vi "Get Challenge Config By Id.vi"(8 "Error In":errorcluster, 11 "VIChallenge Config":T2) -> (0 "Error Out":errorcluster, 2 "Challenge Config":T1, 3 "VIChallenge Config":T2)   [LabVIEW 2013, in "VIChallenge.lvlib"]
uses:
  VIChallenge.lvlib
  Type Defs/VIChallenge Config.ctl
  <vilib>/National Instruments/NI Amazon Web Services (AWS) Toolkit for LabVIEW/SQS/VI Source/AWS SQS Class/AWS_SQS.lvclass
  <vilib>/National Instruments/NI Amazon Web Services (AWS) Toolkit for LabVIEW/AWS Core Lib/VI Source/Typedefs/AWS_AWS Credentials.ctl
  Type Defs/JSON_job.ctl
  <vilib>/addons/database/Connection.llb/Conn ObjectReference.ctl
  Grader/Type Defs/Challenge.ctl
  <vilib>/National Instruments/NI Amazon Web Services (AWS) Toolkit for LabVIEW/AWS Core Lib/VI Source/AWS_Core.lvlib
  <vilib>/addons/database/NI_Database_API.lvlib
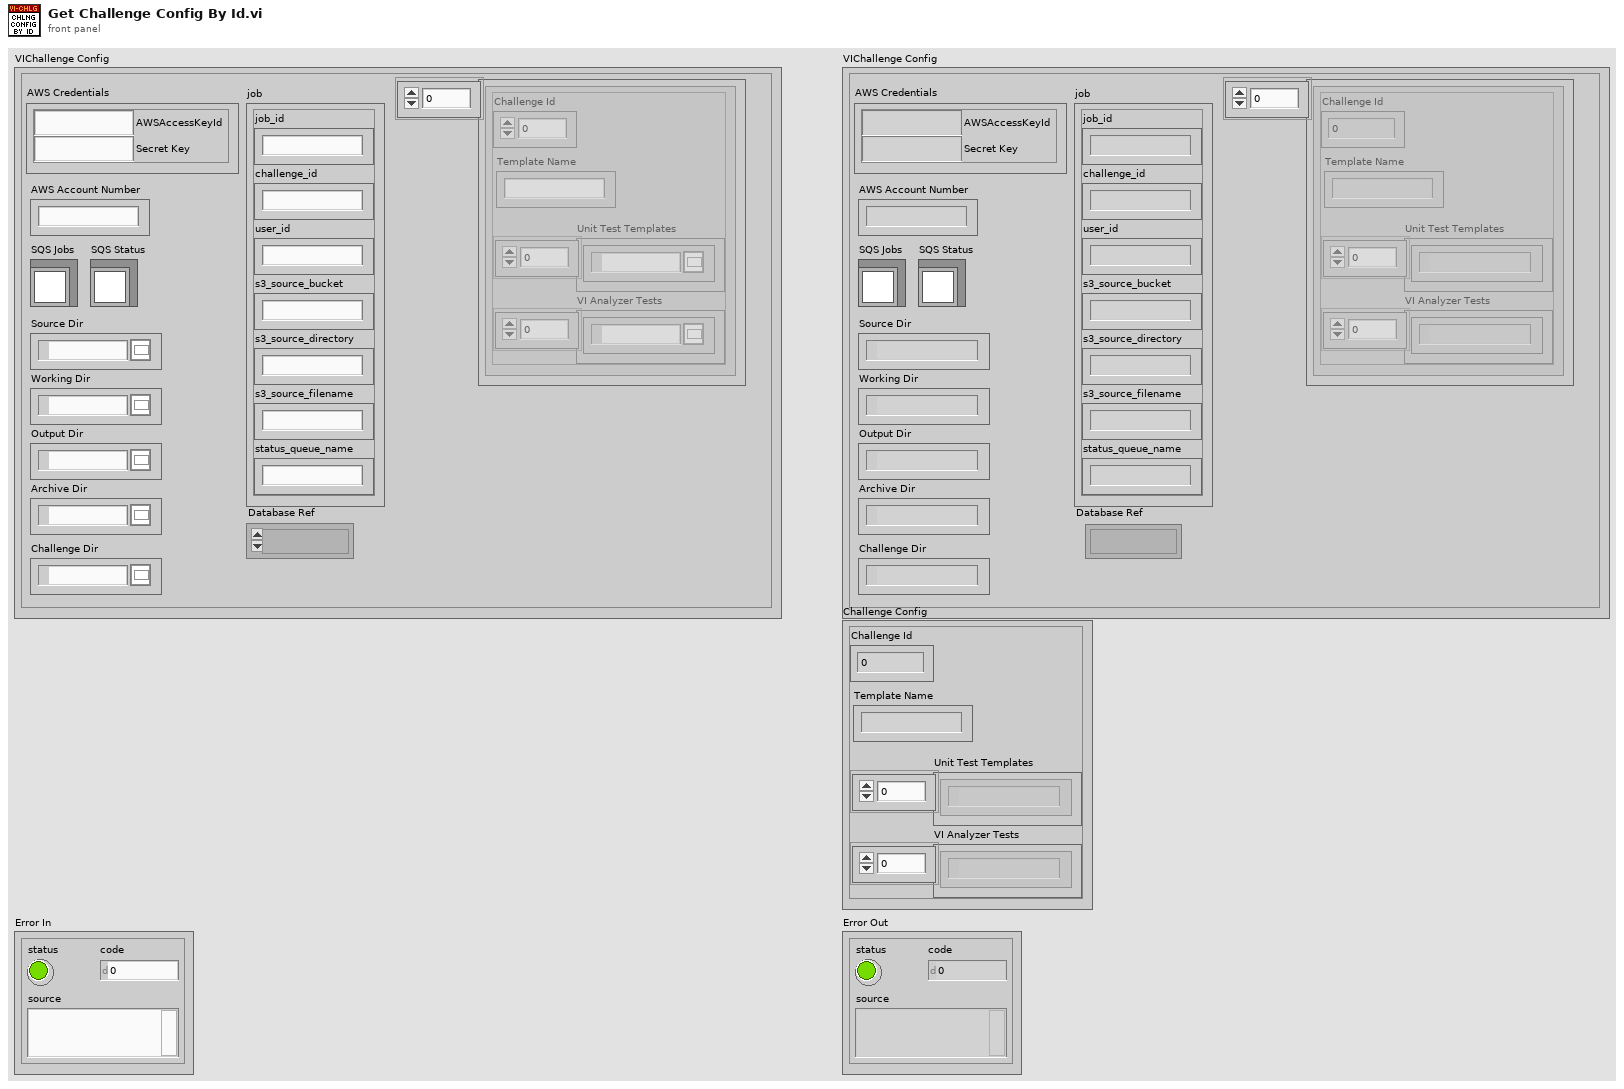
[diagram p1: front panel]
types:
  T1 = typedef "VIChallenge.lvlib/Challenge.ctl" = cluster{"Challenge Id":i32, "Unit Test Templates":path[], "VI Analyzer Tests":path[], "Template Name":string}
  T2 = typedef "VIChallenge.lvlib/VIChallenge Config.ctl" = cluster{"AWS Credentials":T3, "AWS Account Number":string, "SQS Jobs":refnum<class "AWS_SQS.lvclass">, "SQS Status":refnum<class "AWS_SQS.lvclass">, "Source Dir":path, "Working Dir":path, "Output Dir":path, "Archive Dir":path, "job":T4, "Database Ref":T5, "Challenge Dir":path, "Challenges":T1[]}
  T3 = typedef "AWS_Core.lvlib/AWS_AWS Credentials.ctl" = cluster{"AWSAccessKeyId":string, "Secret Key":string}
  T4 = typedef "VIChallenge.lvlib/JSON_job.ctl" = cluster{"job_id":string, "challenge_id":string, "user_id":string, "s3_source_bucket":string, "s3_source_directory":string, "s3_source_filename":string, "status_queue_name":string}
  T5 = typedef "NI_Database_API.lvlib/Conn ObjectReference.ctl" = refnum<k1>
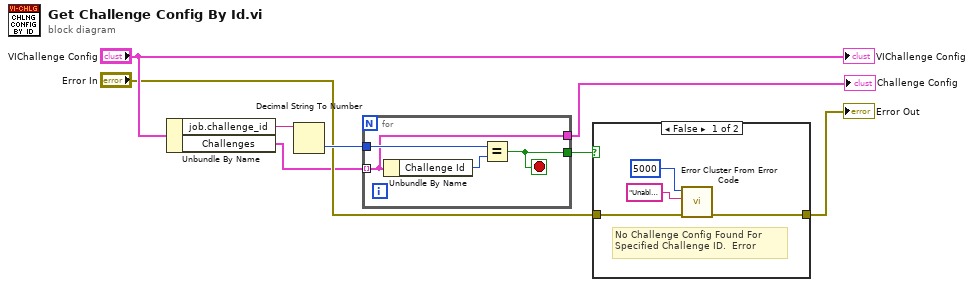
[diagram p0: block diagram]
diagram:
  n1 = Unbundle By Name("VIChallenge Config") -> ("job.challenge_id"=w5:string, "Challenges"=w1:T1[])
  n2 = Decimal String To Number(string=w5) -> (number=w6:i32)  [unwired: 2 in, 1 out]
  n3 = for {
    tunnel: w1 -> [w9] mode=indexing
    tunnel: w6 -> [w11]
    tunnel: [w10] -> w7
    tunnel: [w9] -> w2
    stop <- w10 stop-if-true
    n4 = Unbundle By Name(w9) -> ("Challenge Id"=w12:i32)
    n5 = Equal?(x=w11, y=w12) -> (x = y?=w10:bool)
  }
  "Challenge Config" <- w2
  n6 = case shown="False" w7 {
    tunnel: "Error In" -> [w16 w17]
    tunnel: [w14 w17] -> w8
    frame False {
      # "No Challenge Config Found For \nSpecified Challenge ID.  Error"
      n7 = call <vilib>:"Error Cluster From Error Code.vi"("error in (no error)"=w16, "error message (\"\")"="Unable To Find Challenge Config For Specified Challenge ID." ("error message (\"\")"), "error code (0)"=5000) -> ("error out"=w14:errorcluster)  [unwired: 6 in]
    }
    frame True {
      # "Found Challenge Config\nContinue."
    }
  }
  "Error Out" <- w8
  "VIChallenge Config" <- "VIChallenge Config"
